vi "Update Method Accessors.vi"(8 "error in (no error)":errorcluster, 10 "RPC Method Parameters":T1, 11 "Server class in":refnum<vi>) -> (0 "error out":errorcluster, 3 "Server class out":refnum<vi>)   [LabVIEW 2019, in "gRPC Scripting Tools.lvlib"]
uses:
  gRPC Scripting Tools.lvlib
  TypeDefs/RPC Method Parameters.ctl
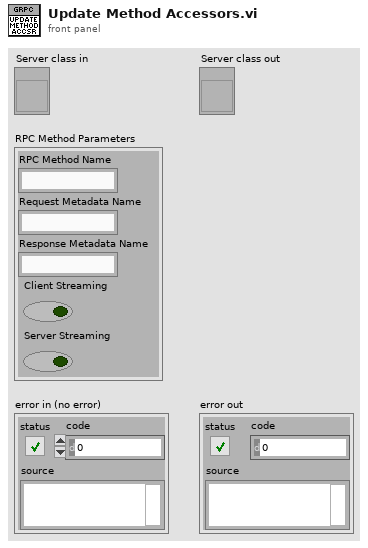
[diagram p1: front panel]
types:
  T1 = typedef "gRPC Scripting Tools.lvlib/RPC Method Parameters.ctl" = cluster{"RPC Method Name":string, "Request Metadata Name":string, "Response Metadata Name":string, "Client Streaming":bool, "Server Streaming":bool}
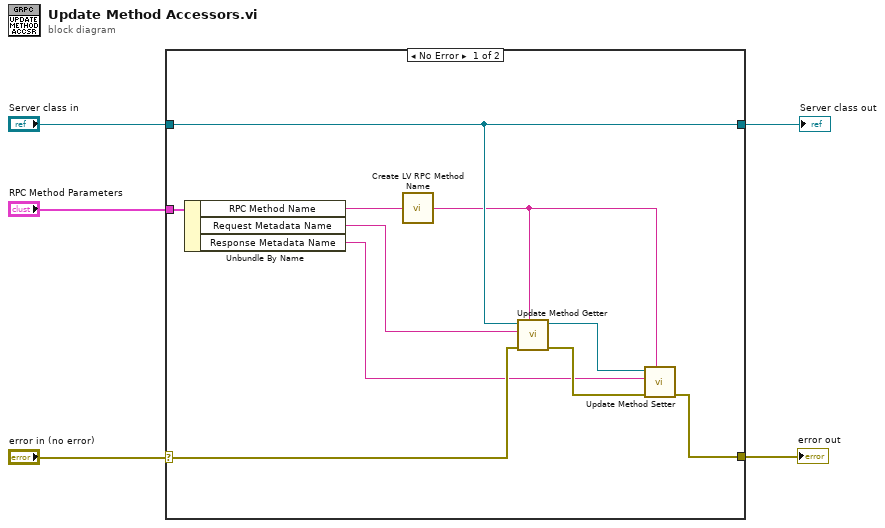
[diagram p0: block diagram]
diagram:
  n1 = case shown="No Error" "error in (no error)" {
    selector: "error in (no error)" -> [w13 w16]
    tunnel: "RPC Method Parameters" -> [w15 _]
    tunnel: "Server class in" -> [w8 w17]
    tunnel: [w8 w17] -> w2
    tunnel: [w9 w16] -> w1
    frame No Error {
      n2 = Unbundle By Name(w15) -> ("RPC Method Name"=w7:string, "Request Metadata Name"=w14:string, "Response Metadata Name"=w10:string)
      n3 = call "Create LV RPC Method Name.vi"("Proto Parser RPC Method Name in"=w7) -> ("LV RPC Method Name out"=w6:string)
      n4 = call "Update Method Getter.vi"("RPC Method Name"=w6, "error in (no error)"=w13, "Request Metadata Name"=w14, "Server class in"=w8) -> ("error out"=w12:errorcluster, "Server class out"=w11:refnum<vi>)  [unwired: 6 in]
      n5 = call "Update Method Setter.vi"("RPC Method Name"=w6, "error in (no error)"=w12, "Response Metadata Name"=w10, "Server class in"=w11) -> ("error out"=w9:errorcluster)  [unwired: 6 in, 1 out]
    }
    frame Error {
    }
  }
  "error out" <- w1
  "Server class out" <- w2
